vi "calculate histogram.vi"(6 "channel no.":i32, 7 "Image Ctrl Ref (as generic class)":refnum<vi>, 8 "Image Array":i16[][](array[numeric]), 11 "Image":T1) -> ()   [LabVIEW 2012]
uses:
  <vilib>/vision/Image Controls.llb/IMAQ Image.ctl
  GFG/GFGfpRefGet.vi
  GFG/GFGbooleanGet.vi
  <vilib>/vision/NI_Vision_Development_Module.lvlib
  GFG/GFG library.lvlib
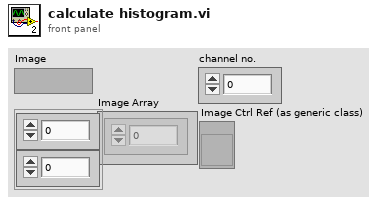
[diagram p1: front panel]
types:
  T1 = typedef "IMAQ Image.ctl" = refnum<image>
  T2 = cluster{"Starting Value":sgl, "Incremental Value":sgl, "Histogram":u32[]}
  T3 = cluster{"WaveformChartRef":refnum<vi>, "DigitalRef":refnum<vi>, "ArrayRef":refnum<vi>, "TabControlRef":refnum<vi>, "EnumRef":refnum<vi>, "RingRef":refnum<vi>, "BooleanRef":refnum<vi>, "KnobRef":refnum<vi>, "SlideRef":refnum<vi>, "PathRef":refnum<vi>, "StringRef":refnum<vi>, "ComboBox":refnum<vi>, "WaveformGraphRef":refnum<vi>}
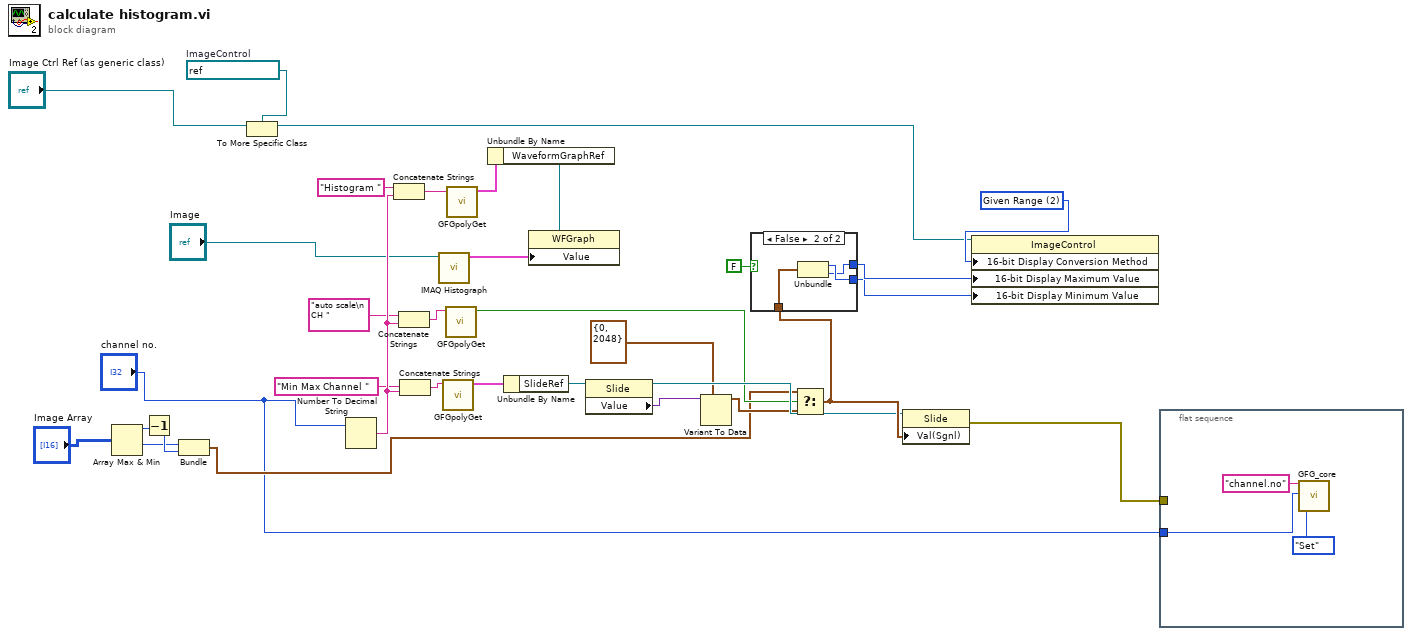
[diagram p0: block diagram]
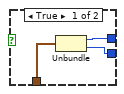
[diagram p2: hidden frame]
diagram:
  w7 = refnum<vi> refnum  # ImageControl
  w15 = u32 2 items=["Full Dynamic", "Downshift", "Given Range", "90% Dynamic", "Given Percent Range"] ("16-bit Display Mapping:Conversion Method")
  n1 = Array Max & Min(array="Image Array") -> (max value=w11:i16, min value=w12:i16)  [unwired: 2 out]
  n2 = Decrement(x=w11) -> (x-1=w13:i16)
  n3 = Bundle(w12, w13) -> (w10:cluster{i16, i16})  [unwired: 1 in]
  n4 = To More Specific Class(target class=w7, reference="Image Ctrl Ref (as generic class)") -> (specific class reference=w6:refnum<vi>)  [unwired: 1 in, 1 out]
  n5 = Number To Decimal String(number="channel no.") -> (decimal integer string=w25:string)  [unwired: 1 in]
  n6 = Concatenate Strings("Histogram " ("string"), w25) -> (w19:string)
  n7 = Concatenate Strings("auto scale\n      CH " ("Variable Name in"), w25) -> (w22:string)
  n8 = Concatenate Strings("Min Max Channel " ("Variable Name in"), w25) -> (w32:string)
  n9 = call "IMAQ Histograph"("Image"="Image") -> ("Histogram Graph"=w16:T2)  [unwired: 7 in, 3 out]
  n10 = call-poly "GFGpolyGet.vi"("Variable Name in"=w32) -> ("output cluster"=w23:T3)  [unwired: 9 in, 1 out]
  n11 = call-poly "GFGpolyGet.vi"("Variable Name in"=w22) -> ("Boolean"=w29:bool)  [unwired: 10 in]
  n12 = call-poly "GFGpolyGet.vi"("Variable Name in"=w19) -> ("output cluster"=w18:T3)  [unwired: 9 in, 1 out]
  n13 = Unbundle By Name(w18) -> ("WaveformGraphRef"=w17:refnum<vi>)
  n14 = Unbundle By Name(w23) -> ("SlideRef"=w26:refnum<vi>)
  n15 = property class="WFGraph"(reference=w17, "Value"=w16) -> ()  [unwired: 1 in, 2 out]
  n16 = property class="Slide"(reference=w26) -> (reference out=w31:refnum<vi>, "Value"=w27:variant)  [unwired: 1 in, 1 out]
  n17 = Variant To Data(type=cluster{i32, i32} {0, 2048} ("channel1"), Variant=w27) -> (data=w30:cluster{i32, i32})  [unwired: 1 in, 1 out]
  n18 = Select(t=w10, s=w29, f=w30) -> (s? t:f=w33:cluster{i32, i32})
  n19 = case shown="False" FALSE {
    tunnel: w33 -> [w36 w39]
    tunnel: [w35 w37] -> w5
    tunnel: [w34 w38] -> w4
    frame True {
      n20 = Unbundle(w36) -> (w35:i32, w34:i32)
    }
    frame False {
      n21 = Unbundle(w39) -> (w38:i32, w37:i32)
    }
  }
  n22 = property class="Slide"(reference=w31, "Val(Sgnl)"=w33) -> (error out=w1:errorcluster)  [unwired: 1 in, 1 out]
  n23 = property class="ImageControl"(reference=w6, "16-bit Display Conversion Method"=w15, "16-bit Display Maximum Value"=w5, "16-bit Display Minimum Value"=w4) -> ()  [unwired: 1 in, 2 out]
  n24 = flat-sequence {
    tunnel: "channel no." -> [w40]
    tunnel: w1 -> [_]
    frame #0 {
      n25 = call "GFG_core.vi"("Variable Name in"="channel.no", "Variant in"=w40, "Action"=enum16{"Init", "Set", "Get"}."Set") -> ()  [unwired: 10 in, 7 out]
    }
  }
